vi "Station Class Server Utility.vi"(8 "error in (no error)":errorcluster, 9 "Action (0: Create)":T1, 10 "Creator Path (=\"\")":path) -> (0 "error out":errorcluster)   [LabVIEW 2018, in "Station.lvclass"]
uses:
  Station.lvclass
  Controls/Server Control.ctl
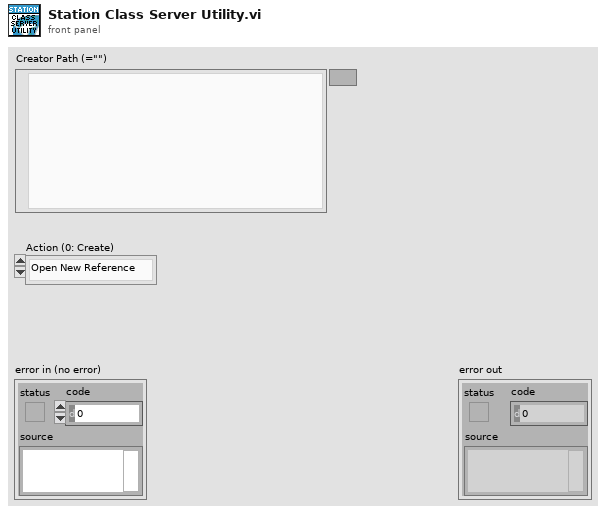
[diagram p1: front panel]
types:
  T1 = typedef "Server Control.ctl" = enum16{"Open New Reference", "Remove Reference", "Kill Server", "Set Station Ref", "Get Station Ref"}
  T2 = enum32{"Invalid", "Standard", "Closed", "Hidden", "Minimized", "Maximized"}
  T3 = cluster{"Action (0: Create)":T1, "Creator Path (=\"\")":path, "Station in":refnum<class "Station.lvclass">}
  T4 = enum32{"Bad", "Idle", "Run top level", "Running"}
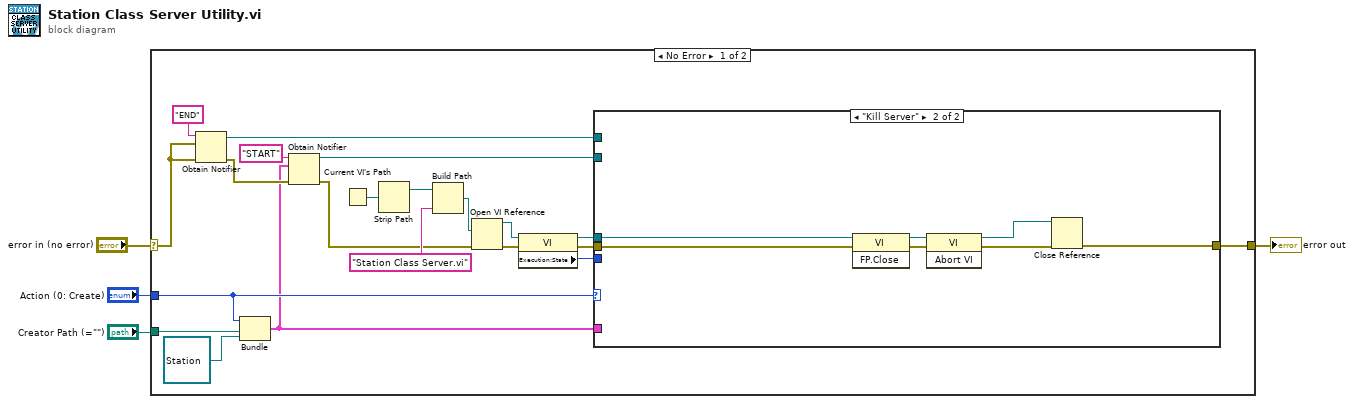
[diagram p0: block diagram]
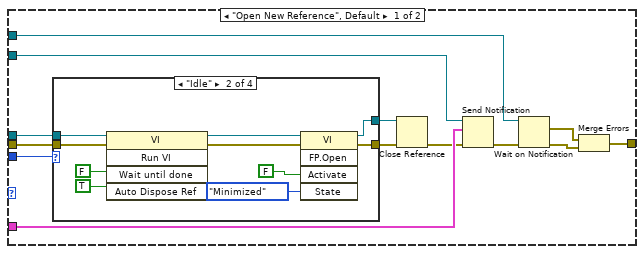
[diagram p2: hidden frame]
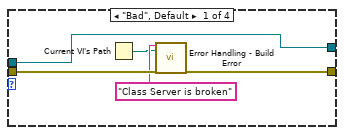
[diagram p3: hidden frame]
diagram:
  n1 = case shown="No Error" "error in (no error)" {
    selector: "error in (no error)" -> [w11 w65]
    tunnel: "Action (0: Create)" -> [w15 _]
    tunnel: "Creator Path (=\"\")" -> [w16 _]
    tunnel: [w6 w65] -> w1
    frame No Error {
      n2 = Obtain Notifier(name (unnamed)="END", notification data type=w11, error in (no error)=w11) -> (notifier out=w8:refnum<notifier>, error out=w14:errorcluster)  [unwired: 1 in, 1 out]
      n3 = Bundle("Action (0: Create)"=w15, "Creator Path (=\"\")"=w16, "Station in"=refnum<class "Station.lvclass"> refnum) -> (w7:T3)  [unwired: 1 in]
      n4 = Obtain Notifier(name (unnamed)="START", notification data type=w7, error in (no error)=w14) -> (notifier out=w9:refnum<notifier>, error out=w10:errorcluster)  [unwired: 1 in, 1 out]
      n5 = Current VI's Path() -> (path=w21:path)
      n6 = Strip Path(path=w21) -> (stripped path=w20:path)  [unwired: 1 out]
      n7 = Build Path(base path=w20, name or relative path="Station Class Server.vi") -> (appended path=w18:path)
      n8 = Open VI Reference(vi path=w18, error in (no error)=w10) -> (vi reference=w24:refnum<vi>, error out=w25:errorcluster)  [unwired: 4 in]
      n9 = property class="VI"(reference=w24, error in=w25) -> (reference out=w17:refnum<vi>, error out=w22:errorcluster, "Execution:State"=w23:T4)
      n10 = case shown="\"Kill Server\"" w15 {
        tunnel: w23 -> [w38 _]
        tunnel: w22 -> [w36 w59]
        tunnel: [w26 w62] -> w6
        tunnel: w17 -> [w37 w58]
        tunnel: w7 -> [w35 _]
        tunnel: w9 -> [w34 _]
        tunnel: w8 -> [w27 _]
        frame "Open New Reference", Default {
          n11 = case shown="\"Idle\"" w38 {
            tunnel: w36 -> [w43 w53 w55 w57]
            tunnel: [w42 w50 w55 w57] -> w33
            tunnel: w37 -> [w39 w45 w54 w56]
            tunnel: [w39 w44 w54 w56] -> w31
            frame "Bad", Default {
              n12 = Current VI's Path() -> (path=w40:path)
              n13 = call "Error Handling - Build Error.vi"("Error Message"="Class Server is broken" ("error message"), "VI Path (calling VI path)"=w40, "error in (no error)"=w43) -> ("error out"=w42:errorcluster)  [unwired: 16 in]
            }
            frame "Idle" {
              n14 = invoke class="VI" method="Run VI"(reference=w45, error in=w53, "Wait until done"=FALSE, "Auto Dispose Ref"=TRUE) -> (reference out=w48:refnum<vi>, error out=w49:errorcluster)  [unwired: 1 in, 3 out]
              n15 = invoke class="VI" method="FP.Open"(reference=w48, error in=w49, "Activate"=FALSE, "State"=T2."Minimized") -> (reference out=w44:refnum<vi>, error out=w50:errorcluster)  [unwired: 1 in, 3 out]
            }
            frame "Run top level" {
            }
            frame "Running" {
            }
          }
          n16 = Close Reference(reference=w31, error in (no error)=w33) -> (error out=w32:errorcluster)
          n17 = Send Notification(notification=w35, notifier=w34, error in (no error)=w32) -> (error out=w28:errorcluster)  [unwired: 1 out]
          n18 = Wait on Notification(notifier=w27, error in (no error)=w28) -> (notification=w29:errorcluster, error out=w30:errorcluster)  [unwired: 2 in, 2 out]
          n19 = Merge Errors(w29, w30) -> (w26:errorcluster)
        }
        frame "Kill Server" {
          n20 = invoke class="VI" method="FP.Close"(reference=w58, error in=w59) -> (reference out=w60:refnum<vi>, error out=w61:errorcluster)  [unwired: 1 in, 1 out]
          n21 = invoke class="VI" method="Abort VI"(reference=w60, error in=w61) -> (reference out=w63:refnum<vi>, error out=w64:errorcluster)  [unwired: 1 in, 1 out]
          n22 = Close Reference(reference=w63, error in (no error)=w64) -> (error out=w62:errorcluster)
        }
      }
    }
    frame Error {
    }
  }
  "error out" <- w1
